vi "RSZVB Delete Power Loss List Single Point.vi"(8 "error in (no error)":errorcluster {"code" format="%.0x"}, 9 "Point (1)":i32=1, 11 "VISA session":refnum<visa-resource-name>) -> (0 "error out":errorcluster {"code" format="%.0x"}, 3 "dup VISA session":refnum<visa-resource-name>)   [LabVIEW 2011]
doc: "This VI deletes a single point no. <List_No> in the power loss list.\n\nRemote-control command(s):\nSOURce<Ch>:POWer<Pt>:CORRection:TCOefficient:DELete<List_No>[:DUMMy]"
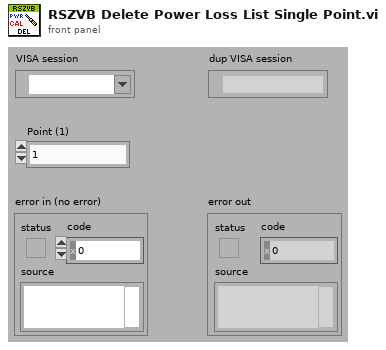
[diagram p1: front panel]
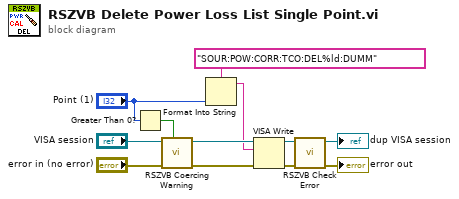
[diagram p0: block diagram]
diagram:
  n1 = Greater Than 0?(x="Point (1)") -> (x > 0?=w9:bool)
  n2 = call "RSZVB Coercing Warning.vi"("In Range?"=w9, "error in (no error)"="error in (no error)", "VISA session"="VISA session") -> ("error out"=w7:errorcluster, "dup VISA session"=w8:refnum<visa-resource-name>)  [unwired: 7 in]
  n3 = Format Into String(format string="SOUR:POW:CORR:TCO:DEL%ld:DUMM", "Point (1)") -> (resulting string=w2:string)  [unwired: 2 in, 1 out]
  n4 = VISA Write(VISA resource name=w8, write buffer=w2, error in (no error)=w7) -> (VISA resource name out=w12:refnum<visa-resource-name>, error out=w11:errorcluster)  [unwired: 1 out]
  n5 = call "RSZVB Check Error.vi"("error in (no error)"=w11, "VISA session"=w12) -> ("error out"=→"error out":errorcluster, "dup VISA session"=→"dup VISA session":refnum<visa-resource-name>)  [unwired: 8 in]
